vi "Percent Span.vi"(8 "error in (no error)":errorcluster, 10 "Input":dbl, 11 "PID in":refnum<class "PID.lvclass">) -> (0 "error out":errorcluster, 2 "% Span":dbl, 3 "PID out":refnum<class "PID.lvclass">)   [LabVIEW 2025]
uses:
  PID.lvclass/PID.ctl
  PID.lvclass
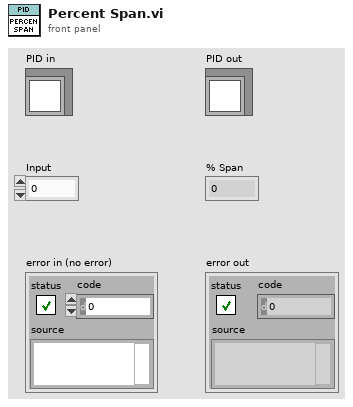
[diagram p1: front panel]
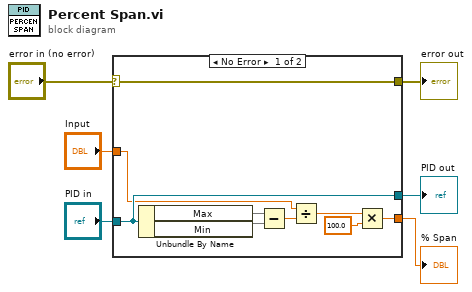
[diagram p0: block diagram]
diagram:
  n1 = case shown="No Error" "error in (no error)" {
    selector: "error in (no error)" -> [w15 w17]
    tunnel: [w15 w17] -> w5
    tunnel: [w14 w16] -> w3
    tunnel: "PID in" -> [w14 w16]
    tunnel: "Input" -> [w11 _]
    tunnel: [w7 _] -> w1
    frame No Error {
      n2 = Unbundle By Name(w14) -> ("Max"=w13, "Min"=w12)
      n3 = Subtract(x=w13, y=w12) -> (x-y=w10:dbl)
      n4 = Divide(x=w11, y=w10) -> (x/y=w9:dbl)
      n5 = Multiply(x=w9, y=100.0) -> (x*y=w7:dbl)
    }
    frame Error {
    }
  }
  "error out" <- w5
  "PID out" <- w3
  "% Span" <- w1
